vi "HUBICACION_POLIGONO.vi"() -> ()   [LabVIEW 2019]
panel:
  out "?":bool
  out "HUBICACION DEL PUNTO 2":string caption="HUBICACION DEL PUNTO"
  out "SUMA DE ANGULOS":dbl
  in  "LONGITUD":dbl[](array[numeric])
  in  "LATITUD":dbl[](array[numeric])=[1.0, 6.0, 14.0, 4.0, 1.0]
  in  "Py":dbl=9.0
  in  "Px":dbl=7.0
  out "POLIGONO LONGITUD VS LATITUD":cluster{"X":dbl[], "Y":dbl[]}[](graph)
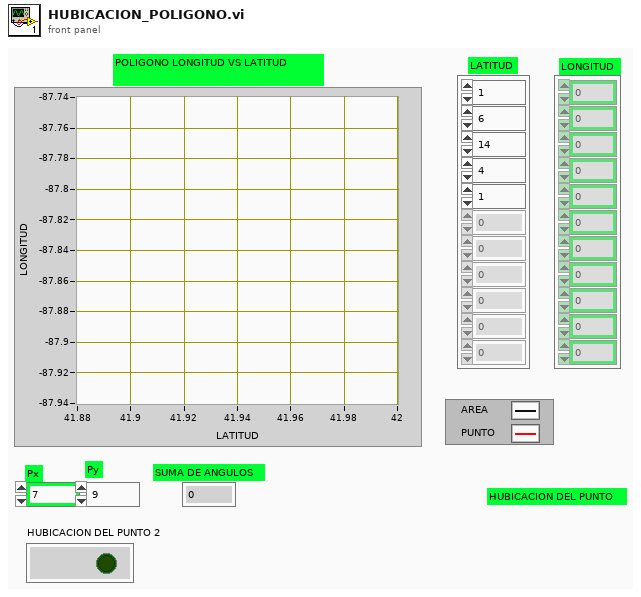
[diagram p1: front panel]
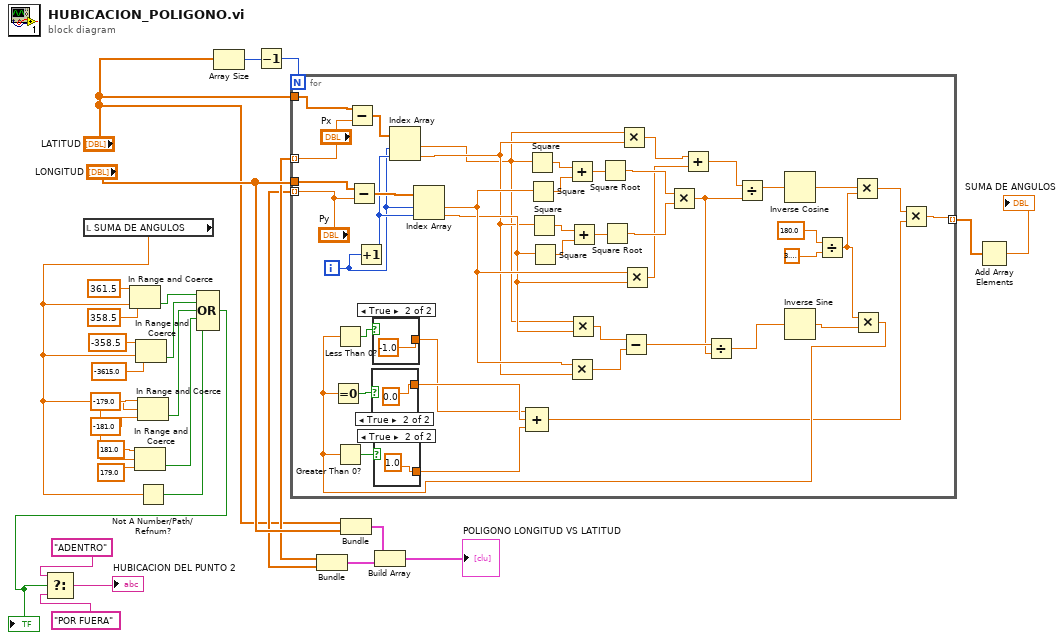
[diagram p0: block diagram]
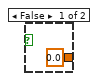
[diagram p2: hidden frame]
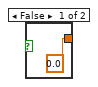
[diagram p3: hidden frame]
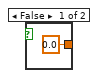
[diagram p4: hidden frame]
diagram:
  n1 = local read "SUMA DE ANGULOS"() -> (w2:dbl)
  n2 = In Range and Coerce(upper limit=361.5, x=w2, lower limit=358.5) -> (In Range?=w17:bool)  [unwired: 1 out]
  n3 = In Range and Coerce(upper limit=181.0, x=w2, lower limit=179.0) -> (In Range?=w5:bool)  [unwired: 1 out]
  n4 = In Range and Coerce(upper limit=-358.5, x=w2, lower limit=-3615.0) -> (In Range?=w14:bool)  [unwired: 1 out]
  n5 = In Range and Coerce(upper limit=-179.0, x=w2, lower limit=-181.0) -> (In Range?=w11:bool)  [unwired: 1 out]
  n6 = Not A Number/Path/Refnum?(number/path/refnum=w2) -> (NaN/Path/Refnum?=w4:bool)
  n7 = Compound Arithmetic op=OR(w17, w14, w11, w5, w4) -> (w3:bool)
  "?" <- w3
  n8 = Select(t="ADENTRO", s=w3, f="POR FUERA") -> (s? t:f=→"HUBICACION DEL PUNTO 2":string)
  n9 = Array Size(array="LATITUD") -> (size(s)=w28:i32)
  n10 = Decrement(x=w28) -> (x-1=w27:i32)
  n11 = for {
    N: w27 -> [_]
    tunnel: "LATITUD" -> [w70]
    tunnel: "LONGITUD" -> [w69]
    tunnel: [w68] -> w21 mode=indexing
    tunnel: ["Px"] -> w26 mode=indexing
    tunnel: ["Py"] -> w25 mode=indexing
    i -> [w67]
    n12 = Subtract(x=w70, y="Px") -> (x-y=w73:dbl[])
    n13 = Subtract(x=w69, y="Py") -> (x-y=w72:dbl[])
    n14 = Increment(x=w67) -> (x+1=w71:i32)
    n15 = Index Array(array=w73, index #1=w67, index #2=w71) -> (element #1=w39:dbl, element #2=w40:dbl)
    n16 = Index Array(array=w72, index #1=w67, index #2=w71) -> (element #1=w42:dbl, element #2=w41:dbl)
    n17 = Square(x=w39) -> (x^2=w64:dbl)
    n18 = Square(x=w42) -> (x^2=w63:dbl)
    n19 = Square(x=w40) -> (x^2=w61:dbl)
    n20 = Square(x=w41) -> (x^2=w60:dbl)
    n21 = Add(x=w64, y=w63) -> (x+y=w62:dbl)
    n22 = Multiply(x=w42, y=w40) -> (x*y=w46:dbl)
    n23 = Multiply(x=w39, y=w41) -> (x*y=w47:dbl)
    n24 = Add(x=w61, y=w60) -> (x+y=w59:dbl)
    n25 = Square Root(x=w62) -> (sqrt(x)=w58:dbl)
    n26 = Square Root(x=w59) -> (sqrt(x)=w57:dbl)
    n27 = Multiply(x=w39, y=w40) -> (x*y=w55:dbl)
    n28 = Subtract(x=w47, y=w46) -> (x-y=w45:dbl)
    n29 = Multiply(x=w42, y=w41) -> (x*y=w56:dbl)
    n30 = Multiply(x=w58, y=w57) -> (x*y=w44:dbl)
    n31 = Add(x=w55, y=w56) -> (x+y=w54:dbl)
    n32 = Divide(x=w45, y=w44) -> (x/y=w43:dbl)
    n33 = Divide(x=w54, y=w44) -> (x/y=w50:dbl)
    n34 = Inverse Cosine(1:w50) -> (0:w53:dbl)
    n35 = Inverse Sine(1:w43) -> (0:w49:dbl)
    n36 = Divide(x=180.0 ("y"), y=3.141592653589793) -> (x/y=w48:dbl)
    n37 = Multiply(x=w53, y=w48) -> (x*y=w38:dbl)
    n38 = Multiply(x=w48, y=w49) -> (x*y=w31:dbl)
    n39 = Equal To 0?(x=w31) -> (x = 0?=w35:bool)
    n40 = Less Than 0?(x=w31) -> (x < 0?=w34:bool)
    n41 = Greater Than 0?(x=w31) -> (x > 0?=w33:bool)
    n42 = case shown="True" w35 {
      tunnel: [0.0 0.0] -> w37
      frame False {
      }
      frame True {
      }
    }
    n43 = case shown="True" w34 {
      tunnel: [0.0 -1.0] -> w36
      frame False {
      }
      frame True {
      }
    }
    n44 = case shown="True" w33 {
      tunnel: [0.0 1.0] -> w32
      frame False {
      }
      frame True {
      }
    }
    n45 = Compound Arithmetic op=ADD(w36, w37, w32) -> (w30:dbl)
    n46 = Multiply(x=w38, y=w30) -> (x*y=w68:dbl)
  }
  n47 = Bundle(w26, w25) -> (w22:cluster{dbl[], dbl[]})  [unwired: 1 in]
  n48 = Bundle("LATITUD"="LATITUD", "LONGITUD"="LONGITUD") -> (w23:cluster{"LATITUD":dbl[], "LONGITUD":dbl[]})  [unwired: 1 in]
  n49 = Build Array(w23, w22) -> (→"POLIGONO LONGITUD VS LATITUD":cluster{"LATITUD":dbl[], "LONGITUD":dbl[]}[])
  n50 = Add Array Elements(numeric array=w21) -> (sum=→"SUMA DE ANGULOS":dbl)
